vi "test Switch Modules To Scan Mode.vi"(8 "error in (no error)":errorcluster, 11 "TestCase in":refnum<class "Scan Engine cRIO 904x-905x System Tests.lvclass">) -> (0 "error out":errorcluster, 3 "TestCase out":refnum<class "Scan Engine cRIO 904x-905x System Tests.lvclass">)   [LabVIEW 2016, in "Scan Engine cRIO 904x-905x System Tests.lvclass"]
uses:
  Scan Engine cRIO 904x-905x System Tests.lvclass
  <vilib>/nisyscfg/Filter Mode.ctl
  <vilib>/nisyscfg/Save Changes (Hardware).vi
  <vilib>/nisyscfg/Close (Resources).vi
  <vilib>/nisyscfg/Close (Filter).vi
  <vilib>/nisyscfg/Close (System).vi
  <vilib>/addons/_JKI Toolkits/VI Tester/TestCase.llb/TestCase.lvclass
  <vilib>/nisyscfg/nisyscfg.lvlib
  <resource>/objmgr/nisysapi.rc
  <resource>/objmgr/nicriosae.rc
  C:/Program Files (x86)/National Instruments/LabVIEW 2016/vi.lib/addons/_JKI Toolkits/VI Tester/TestCase.llb/TestCase.lvclass
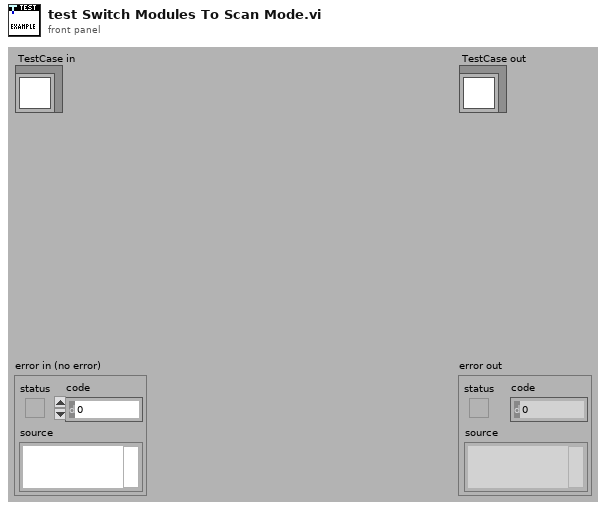
[diagram p1: front panel]
types:
  T1 = cluster{"y":i32, "Devices & Chassis:Bus Specific:cRIO Module Programming Mode":u32}[]
  T2 = typedef "nisyscfg.lvlib/Filter Mode.ctl" = i32
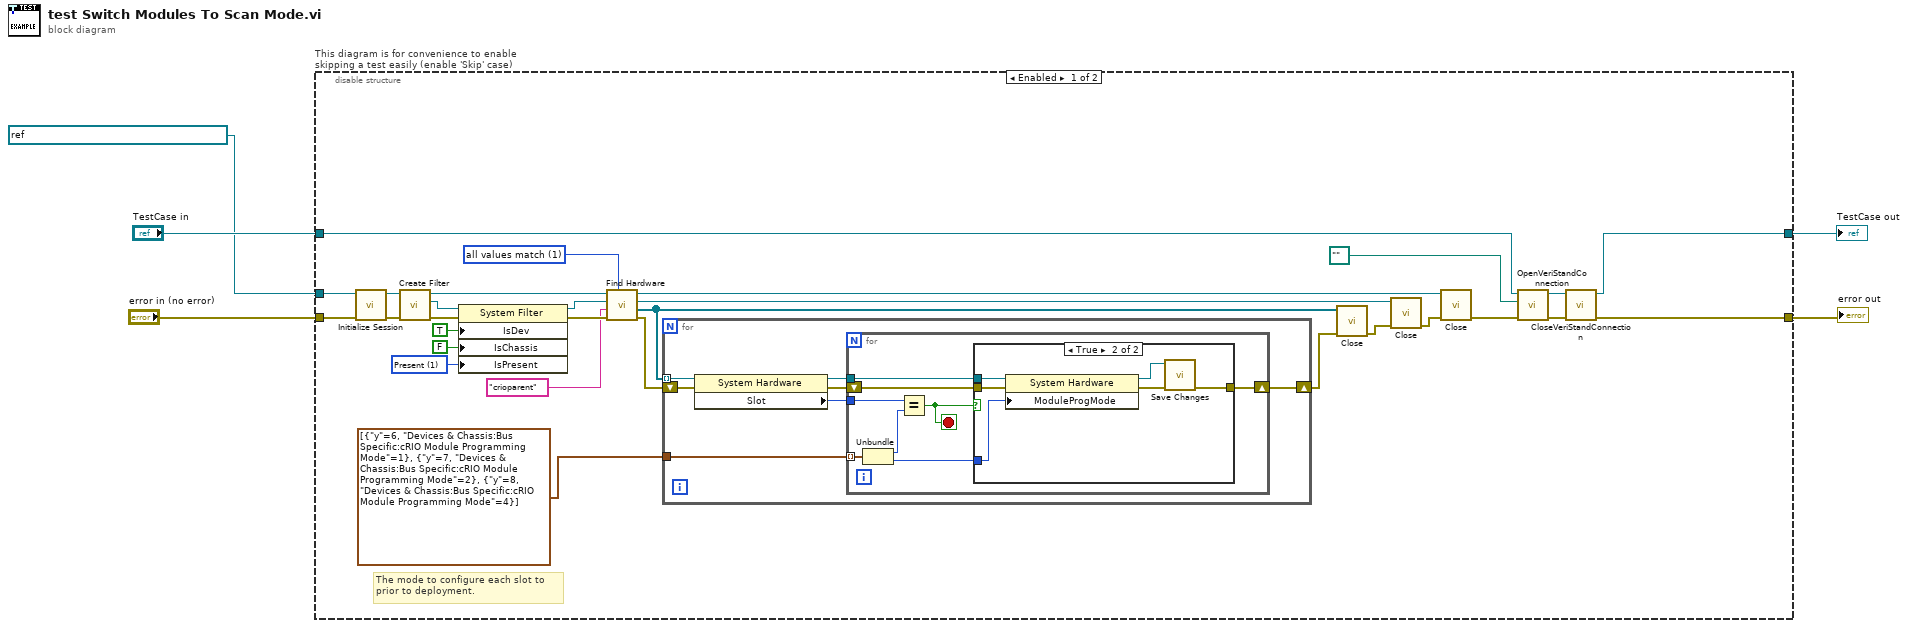
[diagram p0: block diagram]
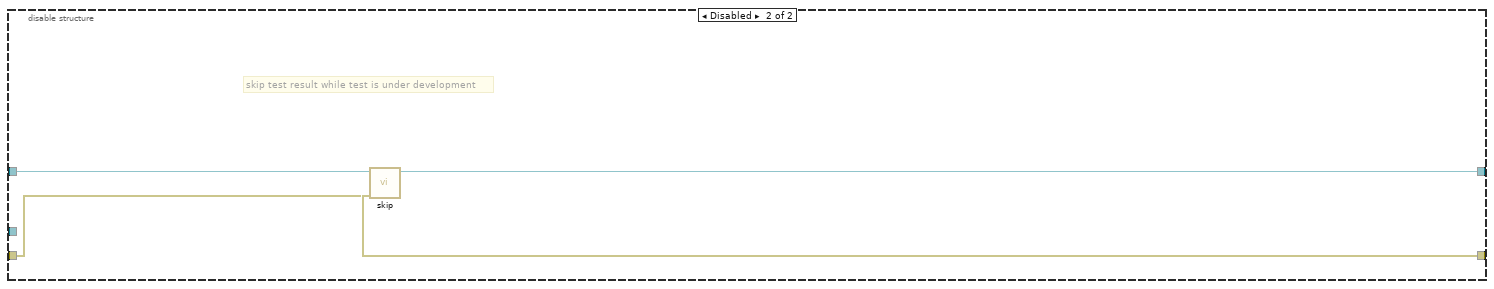
[diagram p3: hidden frame]
diagram:
  n1 = disable-structure "This diagram is for convenience to enable skipping a test easily (enable 'Skip' case)" shown="Enabled" {
    disable-tunnel: "TestCase in" -> [w12 w60]
    disable-tunnel: [w9 w58] -> w2
    disable-tunnel: [w8 w59] -> w4
    disable-tunnel: "error in (no error)" -> [w34 w57]
    disable-tunnel: refnum<k21> "NI-cRIO-9045-01CEEDFB (10.2.64.28)" ("Target (localhost)") -> [w24 _]
    frame Enabled {
      w20 = 1 items=["Initializing"=-2, "Unknown"=-1, "Not Present"=0, "Present"=1] ("Devices & Chassis:Is Present")
      w25 = T2 1 items=["all values match"=1, "any value matches"=2, "values do not match"=3, "all properties exist"=4] ("filter mode (all values match)")
      # "The mode to configure each slot to\nprior to deployment."
      n2 = call <vilib>:"Initialize Session.vi"("error in (no error)"=w34, "Target (localhost)"=w24) -> ("error out"=w26:errorcluster, "Session out"=w27:refnum<k21>)  [unwired: 8 in]
      n3 = call <vilib>:"Create Filter.vi"("error in (no error)"=w26, "Session in"=w27) -> ("error out"=w33:errorcluster, "Filter out"=w32:refnum<k20>, "Session out"=w31:refnum<k21>)  [unwired: 7 in]
      n4 = property class="System Filter"(reference=w32, error in=w33, "IsDev"=TRUE ("Is Chassis"), "IsChassis"=FALSE ("Is Chassis"), "IsPresent"=w20) -> (reference out=w29:refnum<k20>, error out=w30:errorcluster)
      n5 = call <vilib>:"Find Hardware.vi"("Filter Mode (all values match)"=w25, "error in (no error)"=w30, "Experts"="crioparent", "Filter in"=w29, "Session in"=w31) -> ("error out"=w19:errorcluster, "Resources out"=w18:refnum<k20>[], "Filter out"=w23:refnum<k20>, "Session out"=w14:refnum<k21>)  [unwired: 3 out]
      n6 = for {
        tunnel: w18 -> [w40] mode=indexing
        shift-right: [w35] -> w15
        shift-left: w19 -> [w41]
        tunnel: T1 [{"y"=6, "Devices & Chassis:Bus Specific:cRIO Module Programming Mode"=1}, {"y"=7, "Devices & Chassis:Bus Specific:cRIO Module Programming Mode"=2}, {"y"=8, "Devices & Chassis:Bus Specific:cRIO Module Programming Mode"=4}] ("output cluster") -> [w38]
        n7 = property class="System Hardware"(reference=w40, error in=w41) -> (reference out=w37:refnum<k20>, error out=w36:errorcluster, "Slot"=w39:i32)
        n8 = for {
          tunnel: w39 -> [w49]
          tunnel: w38 -> [w48] mode=indexing
          tunnel: w37 -> [w45]
          shift-right: [w43] -> w35
          shift-left: w36 -> [w44]
          stop <- w42 stop-if-true
          n9 = Unbundle(w48) -> ("y"=w47:i32, "Devices & Chassis:Bus Specific:cRIO Module Programming Mode"=w46:u32)
          n10 = Equal?(x=w49, y=w47) -> (x = y?=w42:bool)
          n11 = case shown="True" w42 {
            tunnel: w46 -> [_ w56]
            tunnel: w45 -> [_ w55]
            tunnel: w44 -> [w50 w54]
            tunnel: [w50 w51] -> w43
            frame False {
            }
            frame True {
              n12 = property class="System Hardware"(reference=w55, error in=w54, "ModuleProgMode"=w56) -> (reference out=w53:refnum<k20>, error out=w52:errorcluster)
              n13 = call-poly <vilib>:"Save Changes.vi"("error in (no error)"=w52, "Resource in"=w53) -> ("error out"=w51:errorcluster)  [unwired: 6 in, 3 out]
            }
          }
        }
      }
      n14 = call-poly <vilib>:"Close.vi"("error in (no error)"=w15, "Resources in"=w18) -> ("error out"=w17:errorcluster)  [unwired: 9 in]
      n15 = call-poly <vilib>:"Close.vi"("error in (no error)"=w17, "Filter in"=w23) -> ("error out"=w13:errorcluster)  [unwired: 9 in]
      n16 = call-poly <vilib>:"Close.vi"("error in (no error)"=w13, "Session in"=w14) -> ("error out"=w11:errorcluster)  [unwired: 9 in]
      n17 = call-dynamic "OpenVeriStandConnection.vi"("error in (no error)"=w11, "System Definition File"=path "", "VeriStand Test Case in"=w12) -> ("error out"=w7:errorcluster, "VeriStand Test Case out"=w10:refnum<class "Scan Engine cRIO 904x-905x System Tests.lvclass">)  [unwired: 7 in]
      n18 = call-dynamic "CloseVeriStandConnection.vi"("error in (no error)"=w7, "VeriStand Test Case in"=w10) -> ("error out"=w8:errorcluster, "VeriStand Test Case out"=w9:refnum<class "Scan Engine cRIO 904x-905x System Tests.lvclass">)  [unwired: 8 in]
    }
    frame Disabled {
      # "skip test result while test is under development"
      n19 = call <vilib>:"skip.vi"("error in (no error)"=w57, "TestCase in"=w60) -> ("error out"=w59:errorcluster, "TestCase out"=w58:refnum<class "Scan Engine cRIO 904x-905x System Tests.lvclass">)  [unwired: 8 in]
    }
  }
  "error out" <- w4
  "TestCase out" <- w2
